vi "数值簇元素排列适应窗格.vi"(8 "error in (no error)":errorcluster caption="错误输入（无错误）", 11 "引用":refnum<vi>) -> (0 "error out":errorcluster caption="错误输出")   [LabVIEW 2018]
uses:
  <vilib>/Utility/miscctls.llb/LVPositionTypeDef.ctl
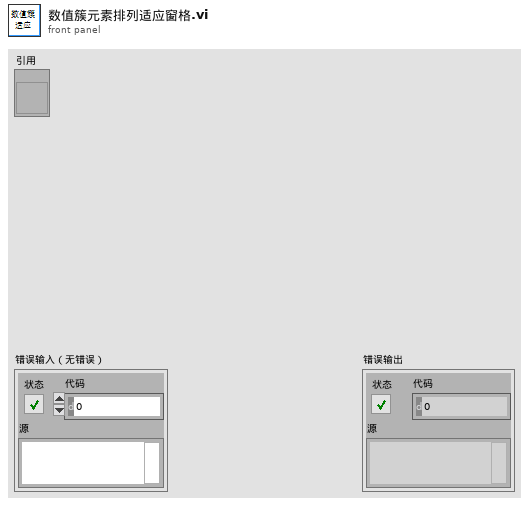
[diagram p1: front panel]
types:
  T1 = typedef "LVPositionTypeDef.ctl" = cluster{"Left":i32, "Top":i32}
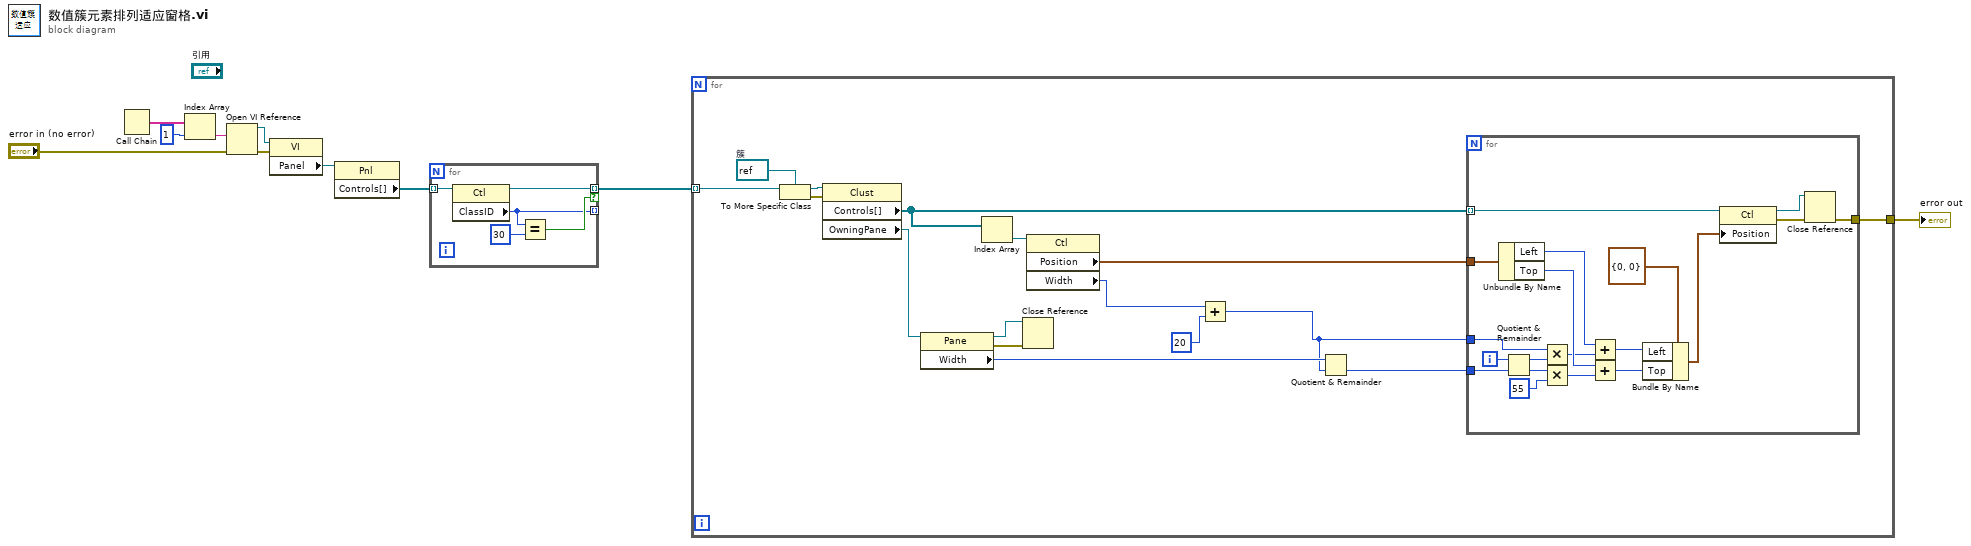
[diagram p0: block diagram]
diagram:
  n1 = Call Chain() -> (call chain=w10:string[])
  n2 = Index Array(array=w10, index=1 ("索引")) -> (element=w6:string)
  n3 = Open VI Reference(vi path=w6, error in (no error)="error in (no error)") -> (vi reference=w1:refnum<vi>, error out=w8:errorcluster)  [unwired: 4 in]
  n4 = property class="VI"(reference=w1, error in=w8) -> ("Panel"=w7:refnum<vi>)  [unwired: 2 out]
  n5 = property class="Pnl"(reference=w7) -> ("Controls[]"=w3:refnum<vi>[])  [unwired: 1 in, 2 out]
  n6 = for {
    tunnel: w3 -> [w15] mode=indexing
    tunnel: [w14] -> w2 mode=indexing if=w12
    tunnel: [w11] -> _ mode=indexing
    n7 = property class="Ctl"(reference=w15) -> (reference out=w14:refnum<vi>, "ClassID"=w11:u32)  [unwired: 1 in, 1 out]
    n8 = Equal?(x=w11, y=u32 30) -> (x = y?=w12:bool)
  }
  n9 = for {
    tunnel: w2 -> [w18] mode=indexing
    tunnel: [w19] -> w4
    w29 = refnum<vi> refnum  # 簇
    n10 = To More Specific Class(target class=w29, reference=w18) -> (specific class reference=w31:refnum<vi>, error out=w30:errorcluster)  [unwired: 1 in]
    n11 = property class="Clust"(reference=w31, error in=w30) -> ("Controls[]"=w17:refnum<vi>[], "OwningPane"=w20:refnum<vi>)  [unwired: 2 out]
    n12 = property class="Pane"(reference=w20) -> (reference out=w28:refnum<vi>, error out=w27:errorcluster, "Width"=w26:u32)  [unwired: 1 in]
    n13 = Index Array(array=w17) -> (element=w25:refnum<vi>)  [unwired: 1 in]
    n14 = Close Reference(reference=w28, error in (no error)=w27) -> ()  [unwired: 1 out]
    n15 = property class="Ctl"(reference=w25) -> ("Position"=w24:T1, "Width"=w16:u32)  [unwired: 1 in, 2 out]
    n16 = Add(x=w16, y=u32 20 ("x")) -> (x+y=w21:u32)
    n17 = Quotient & Remainder(x=w26, y=w21) -> (floor(x/y)=w23:u32)  [unwired: 1 out]
    n18 = for {
      tunnel: w17 -> [w32] mode=indexing
      tunnel: [w48] -> w19
      tunnel: w24 -> [w47]
      tunnel: w23 -> [w40]
      tunnel: w21 -> [w35]
      i -> [w39]
      n19 = Unbundle By Name(w47) -> ("Left"=w42:i32, "Top"=w41:i32)
      n20 = Quotient & Remainder(x=w39, y=w40) -> (x-y*floor(x/y)=w38:u32, floor(x/y)=w37:u32)
      n21 = Multiply(x=w35, y=w38) -> (x*y=w36:u32)
      n22 = Multiply(x=w37, y=u32 55) -> (x*y=w34:u32)
      n23 = Add(x=w42, y=w36) -> (x+y=w44:u32)
      n24 = Add(x=w41, y=w34) -> (x+y=w43:u32)
      n25 = Bundle By Name(cluster=T1 {"Left"=0, "Top"=0} ("位置"), "Left"=w44, "Top"=w43) -> (w45:T1)
      n26 = property class="Ctl"(reference=w32, "Position"=w45) -> (reference out=w50:refnum<vi>, error out=w49:errorcluster)  [unwired: 1 in]
      n27 = Close Reference(reference=w50, error in (no error)=w49) -> (error out=w48:errorcluster)
    }
  }
  "error out" <- w4
